vi "Culver Drive.vi"(6 "Toggle Throttle":bool, 7 "Toggle R":bool, 8 "Sensitivity":ext format="%#.6f", 9 "Throttle":dbl(knob) scale=-1.0..1.0, 10 "Y":dbl(knob) step=0.1 scale=-1.0..1.0, 11 "X":dbl(knob) step=0.1 scale=-1.0..1.0) -> (2 "Right Motor":ext, 3 "Left Motor":ext)   [LabVIEW 2014]
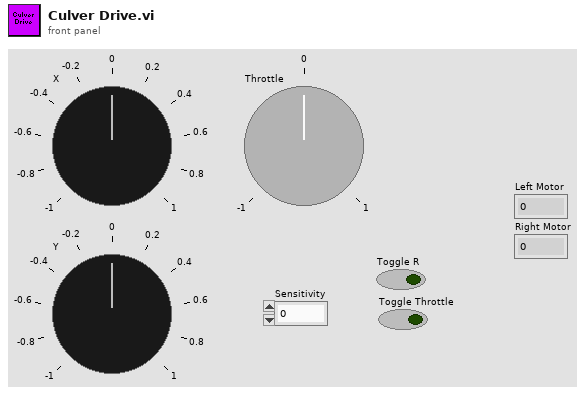
[diagram p1: front panel]
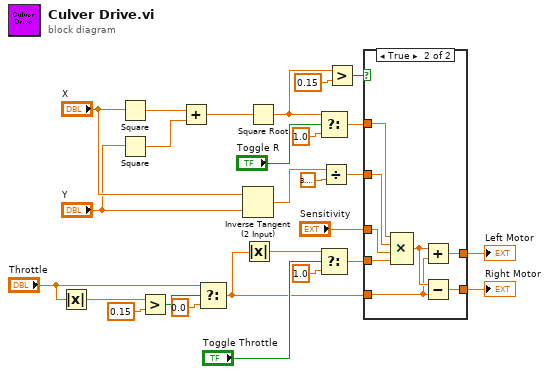
[diagram p0: block diagram]
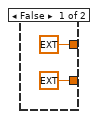
[diagram p2: hidden frame]
diagram:
  n1 = Absolute Value(x="Throttle") -> (abs(x)=w2:dbl)
  n2 = Square(x="X") -> (x^2=w25:dbl)
  n3 = Square(x="Y") -> (x^2=w26:dbl)
  n4 = Greater?(x=w2, y=0.15) -> (0:w4:bool)
  n5 = Add(x=w25, y=w26) -> (x+y=w24:dbl)
  n6 = Select(t="Throttle", s=w4, f=0.0) -> (s? t:f=w5:dbl)
  n7 = Inverse Tangent (2 Input)(1:"Y", 2:"X") -> (0:w22:dbl)
  n8 = Absolute Value(x=w5) -> (abs(x)=w12:dbl)
  n9 = Square Root(x=w24) -> (sqrt(x)=w7:dbl)
  n10 = Select(t=w7, s="Toggle R", f=1.0) -> (s? t:f=w14:dbl)
  n11 = Select(t=w12, s="Toggle Throttle", f=1.0) -> (s? t:f=w13:dbl)
  n12 = Divide(x=w22, y=3.141592653589793) -> (x/y=w21:dbl)
  n13 = Greater?(x=w7, y=0.15) -> (0:w17:bool)
  n14 = case shown="True" w17 {
    tunnel: w14 -> [_ w37]
    tunnel: w13 -> [_ w36]
    tunnel: "Sensitivity" -> [_ w35]
    tunnel: w21 -> [_ w34]
    tunnel: [ext 0.0 w32] -> w19
    tunnel: [ext 0.0 w31] -> w18
    tunnel: w5 -> [_ w30]
    frame False {
    }
    frame True {
      n15 = Compound Arithmetic op=MULTIPLY(w37, w34, w35, w36) -> (w33:ext)
      n16 = Add(x=w33, y=w30) -> (x+y=w32:ext)
      n17 = Subtract(x=w33, y=w30) -> (x-y=w31:ext)
    }
  }
  "Left Motor" <- w19
  "Right Motor" <- w18
